vi "Master Setup Re-register Events.vi"(8 "Master/Channel Subpanel Restarted":bool, 9 "Reset Register Events":bool, 11 "Pattern Label":T1 items=["Channel Setup (0)", "PID Setup (1)", "Filter Setup (2)", "~Reserved Old CAN Msgs (3)", "~Reserved Old CAN1 (4)", "~Reserved Old CAN2 (5)", "Digital Inputs Setup (6)", "Digital Outputs Setup (7)", "Logging 1 Setup (8)", "Logging 2 Setup (9)", "Logging 3 Setup (10)", "Setpoint Setup (11)", "Test Series Setup (12)", "Graph Setup (13)", "System Configure (14)", "Header (15)", "Profile Manager (16)", "Post-Mortem Logging (17)", "High-Speed Data (18)", "Statistic Channel Setup (19)", "Ramp Channel Setup (20)", "ETAS INCA Channel Setup (21)", "ETC ECCS Transducer Setup (22)", "ETC ECCS Test Setup (23)", "AVL AK Smoke Meter Setup (24)", "Triggers Setup (25)", "Alarm Limits Setup (26)", "YKWT1 Measurement (27)", "YKWT1 Instrument (28)", "Auto File Settings (29)", "Playback File Setting (30)", "UUT Constants (31)", "UPS Setup (32)", "Differential Channel Setup (33)", "Integral Channel Setup (34)", "Signal Channel Setup (35)", "Calibration Setup (36)", "BNC Setup (37)", "ASAP3 Setup (38)", "Chassis Force Calculations (39)", "Chassis Teststand Losses (40)", "Chassis Vehicle Losses (41)", "Formula Channels (42)", "ASAP3 Map Coords Setup (43)", "Digital Controls Setup (44)", "Push Buttons Setup (45)", "Sliders Setup (46)", "~Reserved~ (47)", "Email Setup (48)", "Timer Setup (49)", "Unit Conversion Setup (50)", "Visible Channels (51)", "Main Display Setup (52)", "Message Display Setup (53)", "Input Display Setup (54)", "Unico Parameter Downloads (55)", "Flow Meter Setup (56)", "Channel Zero Offset (57)", "YKWT2 Measurement (58)", "YKWT2 Instrument (59)", "~Reserved Old CAN3 (60)", "CAS Setup (61)", "Accumulation Channel Setup (62)", "Valvetrain Dynamics Setup (63)", "CCP Setup (64)", "System Log Setup (65)", "Throttle Controller (66)", "RE Shifter (67)", "Main Display (68)", "~Reserved~ (69)", "FlexRay (70)", "YKWT3 Measurement (71)", "YKWT3 Instrument (72)", "CAN XNET API (73)"]) -> (3 "Re-register Events":bool)   [LabVIEW 2017]
uses:
  Master Setup Pattern Enum.ctl
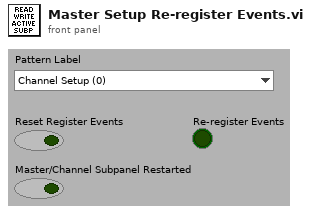
[diagram p1: front panel]
types:
  T1 = typedef "Master Setup Pattern Enum.ctl" = i32
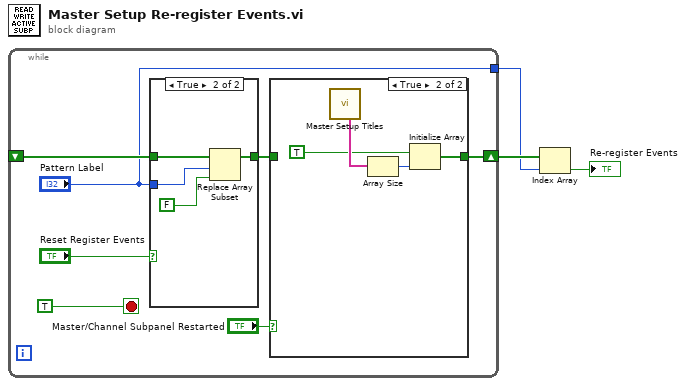
[diagram p0: block diagram]
diagram:
  n1 = while {
    shift-right: [w8] -> w2
    shift-left: _ -> [w7]
    tunnel: ["Pattern Label"] -> w1
    stop <- TRUE stop-if-true
    n2 = case shown="True" "Reset Register Events" {
      tunnel: [w11 w15] -> w6
      tunnel: w7 -> [w11 w14]
      tunnel: "Pattern Label" -> [_ w13]
      frame False {
      }
      frame True {
        n3 = Replace Array Subset(array=w14, new element=FALSE ("new element/subarray"), index=w13) -> (w15:bool[])
      }
    }
    n4 = case shown="True" "Master/Channel Subpanel Restarted" {
      tunnel: [w16 w20] -> w8
      tunnel: w6 -> [w16 _]
      frame False {
      }
      frame True {
        n5 = call "Master Setup Titles.vi"() -> ("Sorted Setup Description"=w19:string[])  [unwired: 6 in, 5 out]
        n6 = Array Size(array=w19) -> (size(s)=w18:i32)
        n7 = Initialize Array(TRUE ("status"), w18) -> (w20:bool[])
      }
    }
  }
  n8 = Index Array(array=w2, index=w1) -> (element=→"Re-register Events":bool)
